vi "write_data_Excel_tab.vi"(2 "text data":string[][](array[string])=[["23", "3/22/2019", "30101566", "DM17-20                  ", "                         ", "Fail", "30", "0.14", "1.375", "934.203", "37.774", "0.339"], ["24", "3/22/2019", "30101566", "DM17-20                  ", "                         ", "Fail", "60", "25.11", "1.413", "935.39", "41.68", "29.618"], ["25", "3/22/2019", "30101566", "DM17-20                  ", "                         ", "Fail", "90", "58.98", "1.444", "936.11", "44.048", "45.383"], ["26", "3/22/2019", "30101566", "DM17-20                  ", "                         ", "Fail", "120", "93.3", "1.473", "936.93", "46.745", "52.783"], ["27", "3/22/2019", "30101566", "DM17-20                  ", "                         ", "Fail", "150", "127.7", "1.502", "937.91", "49.969", "56.68"], ["28", "3/22/2019", "30101566", "DM17-20                  ", "                         ", "Fail", "180", "161.8", "1.53", "938.84", "53.028", "58.751"], ["29", "3/22/2019", "30101566", "DM17-20                  ", "                         ", "Fail", "210", "195.3", "1.558", "939.97", "56.745", "59.692"], ["30", "3/22/2019", "30101566", "DM17-20                  ", "                         ", "Fail", "240", "228.2", "1.584", "941.04", "60.265", "60.027"], ["31", "3/22/2019", "30101566", "DM17-20                  ", "                         ", "Fail", "270", "260.1", "1.61", "942.37", "64.64", "59.834"], ["32", "3/22/2019", "30101566", "DM17-20                  ", "                         ", "Fail", "300", "290.9", "1.635", "943.75", "69.18", "59.307"], ["33", "3/22/2019", "30101566", "DM17-20                  ", "                         ", "Fail", "330", "320.2", "1.66", "945.28", "74.212", "58.452"]], 3 "error in (no error)":errorcluster, 4 "worksheet index (0)":i32, 5 "report in":refnum<class "NI_report.lvclass">=refnum) -> (0 "error out":errorcluster, 1 "report out":refnum<class "NI_report.lvclass">)   [LabVIEW 2017]
uses:
  <vilib>/Utility/NIReport.llb/NI_report.lvclass
  <vilib>/Utility/NIReport.llb/Excel/NI_Excel.lvclass
  <vilib>/addons/_office/excel.llb/Excel Easy Table (str).vi
  <vilib>/addons/_office/NI_ReportGenerationToolkit.lvlib
panel:
  in  "start (0, 0)":cluster{"row":i32, "column":i32}={"row"=1, "column"=0}
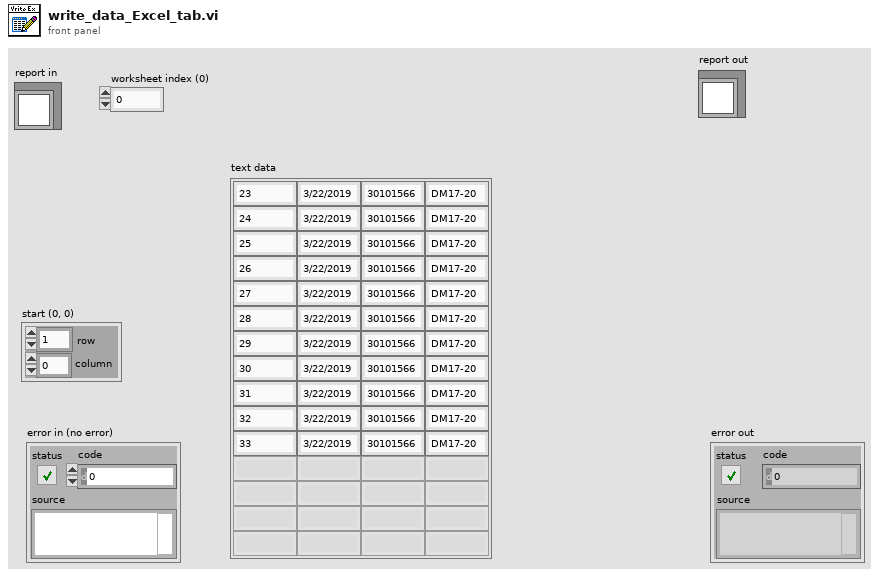
[diagram p1: front panel]
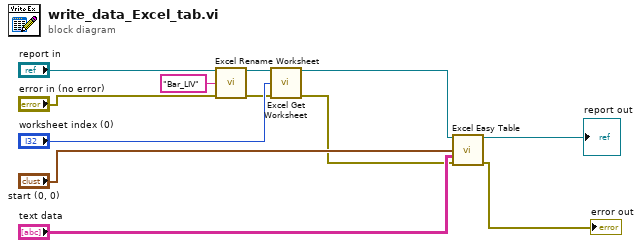
[diagram p0: block diagram]
diagram:
  n1 = call <vilib>:"Excel Rename Worksheet.vi"("report in"="report in", "worksheet name (\"\")"="Bar_LIV" ("worksheet name (\"\")"), "error in (no error)"="error in (no error)") -> ("report out"=w1:refnum<class "NI_report.lvclass">, "error out"=w4:errorcluster)  [unwired: 11 in]
  n2 = call <vilib>:"Excel Get Worksheet.vi"("report in"=w1, "worksheet index (0)"="worksheet index (0)", "error in (no error)"=w4) -> ("report out"=w11:refnum<class "NI_report.lvclass">, "error out"=w7:errorcluster)  [unwired: 11 out]
  n3 = call-poly <vilib>:"Excel Easy Table.vi"("report in"=w11, "start (0, 0)"="start (0, 0)", "text data"="text data", "error in (no error)"=w7) -> ("report out"=→"report out":refnum<class "NI_report.lvclass">, "error out"=→"error out":errorcluster)  [unwired: 7 in, 3 out]
